vi "Forebrain.vi"() -> ()   [LabVIEW 2012]
doc: "This VI contrains the Forebrain within the Olin Robot Architecture. It must be run first to load the appropriate mission definition files. It contains a finite state machine built around a tabbed Operator interface that will guide an operator through the startup, run shutdown mission sequence. After running it, run the Midbrain and Hindbrain VIS."
panel:
  out "return count":u32
  out "error out":errorcluster
  in  "error in 2":errorcluster
  out "Desired \nVelocity":i16=5
  out "Local\nHeading":i16=90
  out "Ycurrent":dbl format="%#_3g"
  out "Xcurrent":dbl format="%#_3g"
  out "Ystart":dbl
  out "Xstart":dbl
  in  "error in":errorcluster
  out "Robot Live":bool
  in  "E-Stop":bool
  in  "Tab":T1(tab)
  out "MissionTime (Min)":dbl(knob) scale=0.0..10.0
  out "LidarDist":i16
  out "IR Index":i32
  out "BatteryLevel":dbl(slide) scale=6.0..9.0
  out "String Received":string
  out "Send String":string="$B^"
  in  "VISA resource name":refnum<visa-resource-name>="COM10"
  in  "Mode":i16 min=0 max=99 step=1
  in  "Desired Vel":i16(slide) scale=-9.0..9.0
  in  "Local Head":i16(slide) scale=-180.0..180.0
  out "StartMissionMap":picture
  out "MapDARCheck":picture
  in  "RunRobot":bool
  in  "Tug letter":string="G"
  out "Tug X":i32
  out "Tug Y":i32
  out "Tug H":i32
  out "BS Time Out?":bool
  out "Buoy locations":cluster{"regular expression":string, i32, i32}[](array[cluster])
  out "Valid ?":bool
  out "Battery\nVolts":i16
  out "Base Station data rec'd":string
  out "udp rate":bool
  out "CollisionWarning":bool
  out "DebugMapDAR":picture
  in  "MapDAR Control":T2={"NumberOfBeams"=180, "SensorRange"=500.0, "Noise (0.1 to 1)"=0.0} {"Noise (0.1 to 1)" min=0.0 max=1.0 step=0.1; "SensorRange" min=500.0 max=1500.0 step=100.0; "NumberOfBeams" min=36 max=360 step=2}
  out "MapDAR Data (r:pixel b:degrees)":cluster{"Range":dbl, "Bearing":dbl}[](array[cluster])
  in  "Stop DebugSENSE":bool
  out "MissionMap":picture
  out "Tug position":T3
  out "initialized MDF":T4(array[cluster])
  out "Way Point Index":i32
  out "InitialWaypoint":cluster{"X":i16, "Y":i16}
  in  "Pen Color":u32(colorbox)=15671808
  in  "Select Pen Attributes":T5={"Width"=1, "Style"=enum."Solid"}
  out "Draw??":bool
  in  "WhereAmI?FromBase":T6
  out "(xr,yr)":cluster{"X":dbl, "Y":dbl}
  in  "RobotPosition":T3 {"xrobot" min=0.0 max=1177.0 step=10.0; "yrobot" min=0.0 max=850.0 step=10.0; "heading" min=0.0 max=7.0 step=0.1}
  out "MDF_Original":T4(array[cluster])
  out "WhatAroundMeMap?":cluster{"T":dbl, "Range":dbl, "Bearing":dbl}[](array[cluster])
  out "WayPointAct":dbl[](array[numeric])
  out "SteerAngle":dbl
  out "MissionDefFile":picture
  out "MDF":T4(array[cluster])
  in  "Select Your Behavior":T7(ring)
  out "No. of Waypoints":i32
  in  "Exit Planning":bool
  in  "BoatSpeed for Leg":dbl(slide) min=-9.0 max=9.0 step=1.0 scale=-9.0..9.0
  out "BuildMDF":bool
  out "WayPoint Position":cluster{"X":i32, "Y":i32}
  out "Send String to NXT":string="$B^"
  in  "Behavior Command":T7(ring)
  out "CollisionLight":bool
  out "Where? Manual":T6
  out "ActManual":bool
  in  "Manual Heading":i16(knob) min=-179 max=180 step=5 scale=180.0..-180.0
  out "MWhat?":bool
  out "Where? 2":bool
  out "How? 2":bool
  in  "ManualModeStop":bool
  out "ManualModeMapDAR":picture
  out "ManualMissionMap":picture
  out "Battery":dbl(slide) scale=0.0..8.0
  in  "Manual Vel":dbl(slide) min=-6.0 max=6.0 step=1.0 scale=-6.0..6.0
  out "MissionTime":dbl(knob) scale=0.0..10.0
  out "Heading":cluster{dbl, dbl}(knob)={0.0, 34.390870865624734} scale=180.0..-179.0 scale format="%#_3g"
  out "Speed":i16(knob) scale=-6.0..6.0
  out "Current Behavior":T7(ring)
  out "Robot Position":cluster{"X":dbl, "Y":dbl} {"X" format="%#_3g"; "Y" format="%#_3g"}
  out "Ready":bool
  in  "Pause":bool
  in  "Rerun MDF":bool
  out "CollisionLight 2":bool
  out "Act":bool
  out "Neo-C":bool
  out "How?":bool
  out "What?":bool
  out "A Heading":cluster{dbl, dbl}(knob)={0.0, 34.390870865624734} scale=180.0..-180.0
  out "A Speed":dbl(knob) scale=-9.0..9.0
  out "AutoBattery":dbl(slide) scale=0.0..8.0
  out "AutoModeLIDAR":picture
  out "AutoMissionMap":picture
  in  "RunAutoMode":bool
  out "MissionTimeAuto":dbl(knob) scale=0.0..60.0
  out "Where?":bool
  # "To run\nrobot,\nclick\narrow\nabove\n\nRun Robot button must be on"
  # "Operation Directions\n\n1)Click on Startup&\nShutdown tab.\n2) Click on Run \nArrow on menubar.\nRun Forebrain,\nvis from the project\nexplorer.\n3) Select a mssion \nmap file when asked.\n4) Check robot is \nfully operational on\nStartup tab.\n5) Debug with debug\ntabs as required.\n6) Select ManualMode\ntab and test drive \nrobot.\n7) Select PlanMission\ntab and set up \nmission.\n8) Go to AutoMode\ntab and run mission."
  # "Turns off drive\nmotors"
  # "Enter Olin Test  Pool"
  # "Xbee Com Port"
  # "xBee\"Send String\" (mode, desired velocity, local heading)"
  # "(Type in Tug Letter  L T G P  (look at boat cradle)"
  # "Should be on to\nrun"
  # "BoatG,X,Y,H,BoatT,X,Y,H,BoatP,X,Y.H,BoatL,X,Y,H,BuoyA,X,Y,BuoyB,X,Y,BuoyC,X,Y,BuoyD,X,Y,Time(hours,Min,Sec)"
  # "To stop  program \nturn off here"
  # "Use this tab\nto explore\nLIDAR\ndata and \noperation"
  # "Set\nNumberOfBeams\nSensorRange\nNoise\nto\nview\nsimulated\nsensor\ndata"
  # "Turn Debug Sim \nto leave this\ntab--->"
  # "This tab will auto\nreturn to Startup \nin 2 seconds"
  # "Clean up interface and make more useful for debugging behaviors"
  # "Build out interface and make more useful for debugging act"
  # "This tab will auto\nreturn to Startup \nin 2 seconds"
  # "Directions:\n1) Select Robot Behavior for each mission leg.\n2) Select Robot Speed for leg.\n3) Click on robots current location for first waypoint.\n4) Hold down button and drag to next\nwaypoint. Click on next leg waypoint.\n5) Hold mouse button down and drag to \nnext waypoint. \n6) Click on next waypoint. Repeat for full mission.\n7) MDF will store up to 20 waypoints."
  # "Remember to\nset boat\nleg speed !"
  # "Please Adjust Scroll Barrs in Tug Off Mode to Prevent  Extra Lines Being Drawn"
  # "\"Send String\" (mode, desired velocity, local heading)"
  # "Press to stop and return to StartUp"
  # "Open MidBrain\nArbiter to see\nBrain Waves"
  # "AutoMode\nAutomatically \nReturns to \nStartUp Mode"
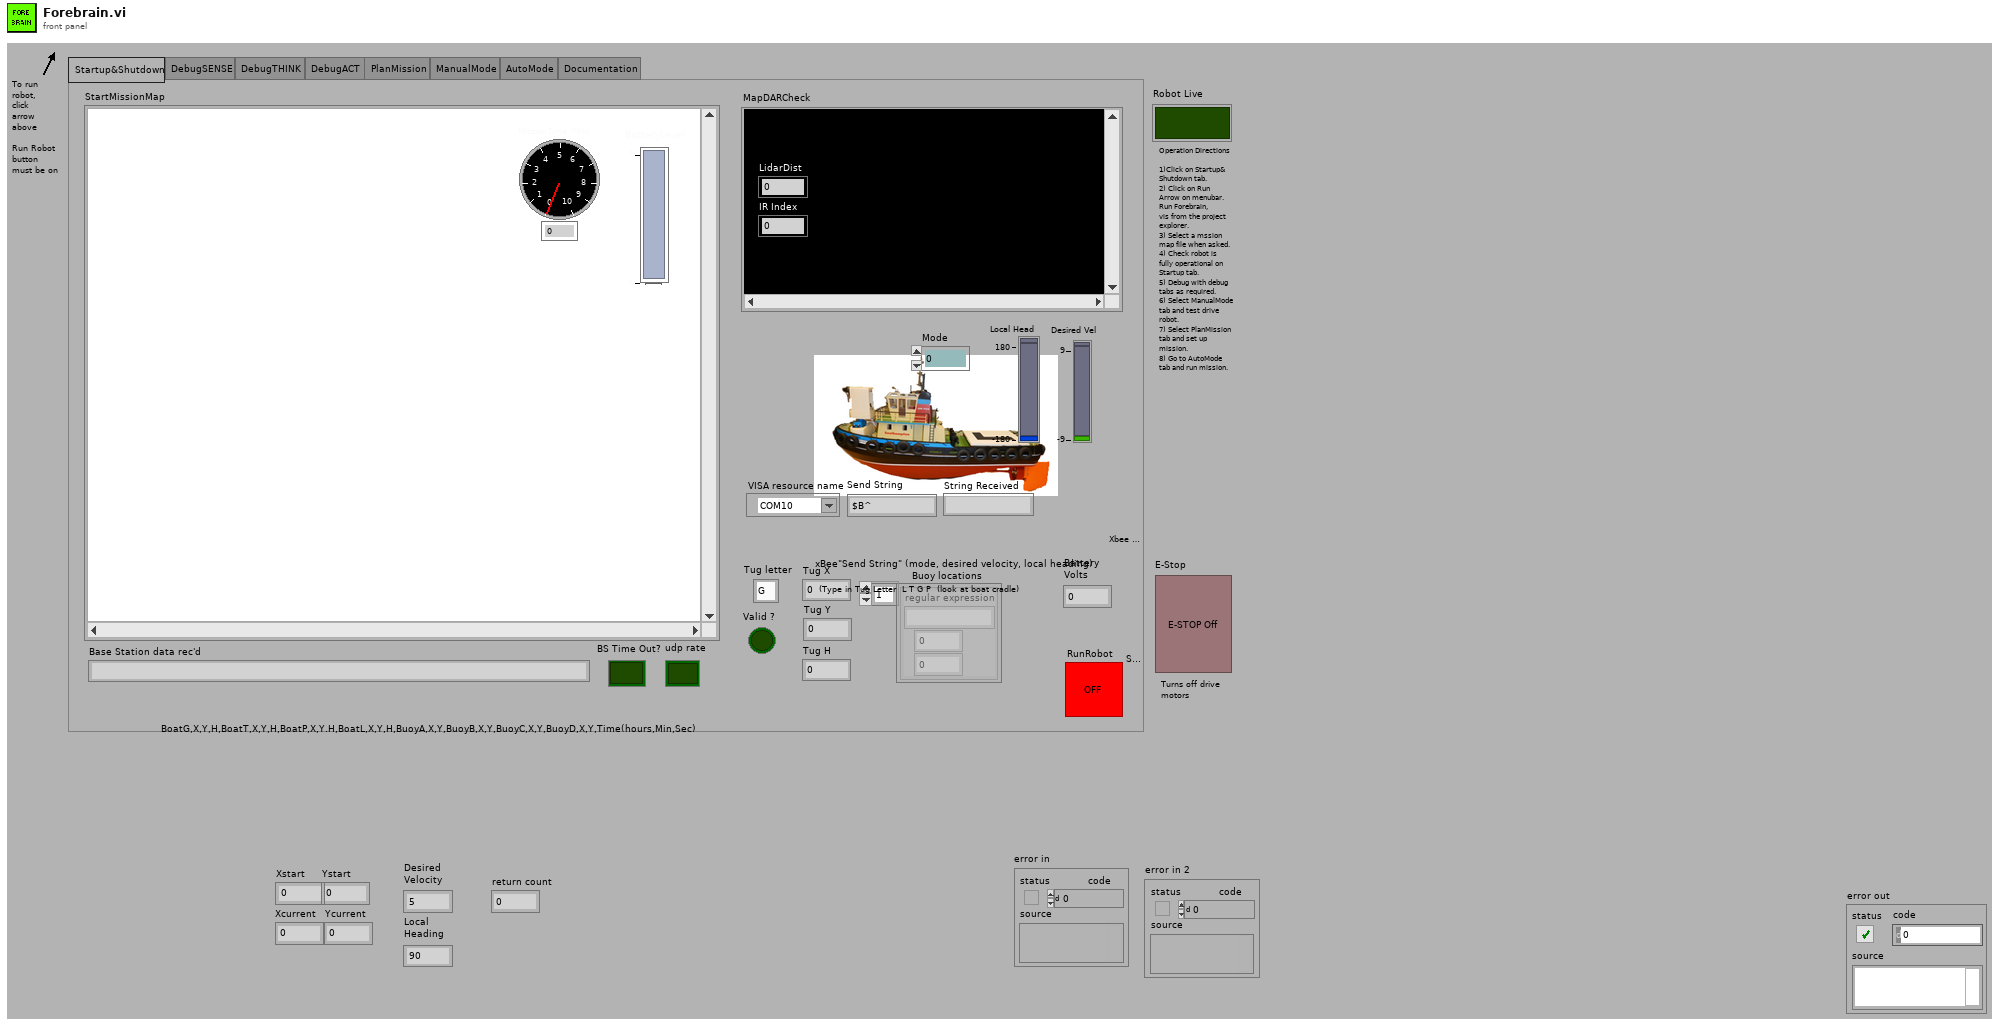
[diagram p1: front panel]
types:
  T1 = enum32{"Startup&Shutdown", "DebugSENSE", "DebugTHINK", "DebugACT", "PlanMission", "ManualMode", "AutoMode", "Documentation"}
  T2 = cluster{"NumberOfBeams":i32, "SensorRange":dbl, "Noise (0.1 to 1)":dbl}
  T3 = cluster{"xrobot":dbl, "yrobot":dbl, "heading":dbl}
  T4 = cluster{"Status":enum16{"Past", "Current", "Future"}, "x":dbl, "y":dbl, "z":dbl, "Vel":dbl, "Dwell Time":dbl, "BehCom":enum16{"Tug Off", "Manual Mode", "Goto WayPoint", "Back Up", "Circle", "Left Wall Follow", "Right Wall Follow", "Hunt"}, "Expand1":dbl, "Expand2":dbl, "Expand3":dbl}[]
  T5 = cluster{"Width":u16, "Style":enum32{"Solid", "Dash", "Dot", "DashDot", "DashDotDot"}}
  T6 = cluster{"T":dbl, "X":dbl, "Y":dbl, "Direction":dbl}
  T7 = enum16{"Tug Off", "Manual Mode", "Goto WayPoint", "Back Up", "Circle", "Left Wall Follow", "Right Wall Follow", "Hunt"}
  T8 = cluster{"VelCom":dbl, "BehCom":enum16{"OpenFieldTransit", "P-WallFollow", "S-WallFollow", "LaneFollow", "ManualMode"}}
  T9 = typedef "IMAQ Image.ctl" = refnum<image>
  T10 = typedef "imagedata.ctl" = cluster{"image type":i32, "image depth":i32, "image":u8[], "mask":u8[], "colors":u32[], "Rectangle":cluster{"left":i16, "top":i16, "right":i16, "bottom":i16}}
  T11 = cluster{"Status":enum16{"Past", "Current", "Future"}, "x":dbl, "y":dbl, "z":dbl, "Vel":dbl, "Dwell Time":dbl, "BehCom":enum16{"Tug Off", "Manual Mode", "Goto WayPoint", "Back Up", "Circle", "Left Wall Follow", "Right Wall Follow", "Hunt"}, "Expand1":dbl, "Expand2":dbl, "Expand3":dbl}
  T12 = typedef "LVMouseTypeDef.ctl" = cluster{"Mouse Position":cluster{"X":i32, "Y":i32}, "Mouse Modifiers":cluster{"Button Down":bool, "Shift Mod":bool, "Menu Mod":bool, "Option Mod":bool}}
  T13 = cluster{"regular expression":string, i32, i32, i32}
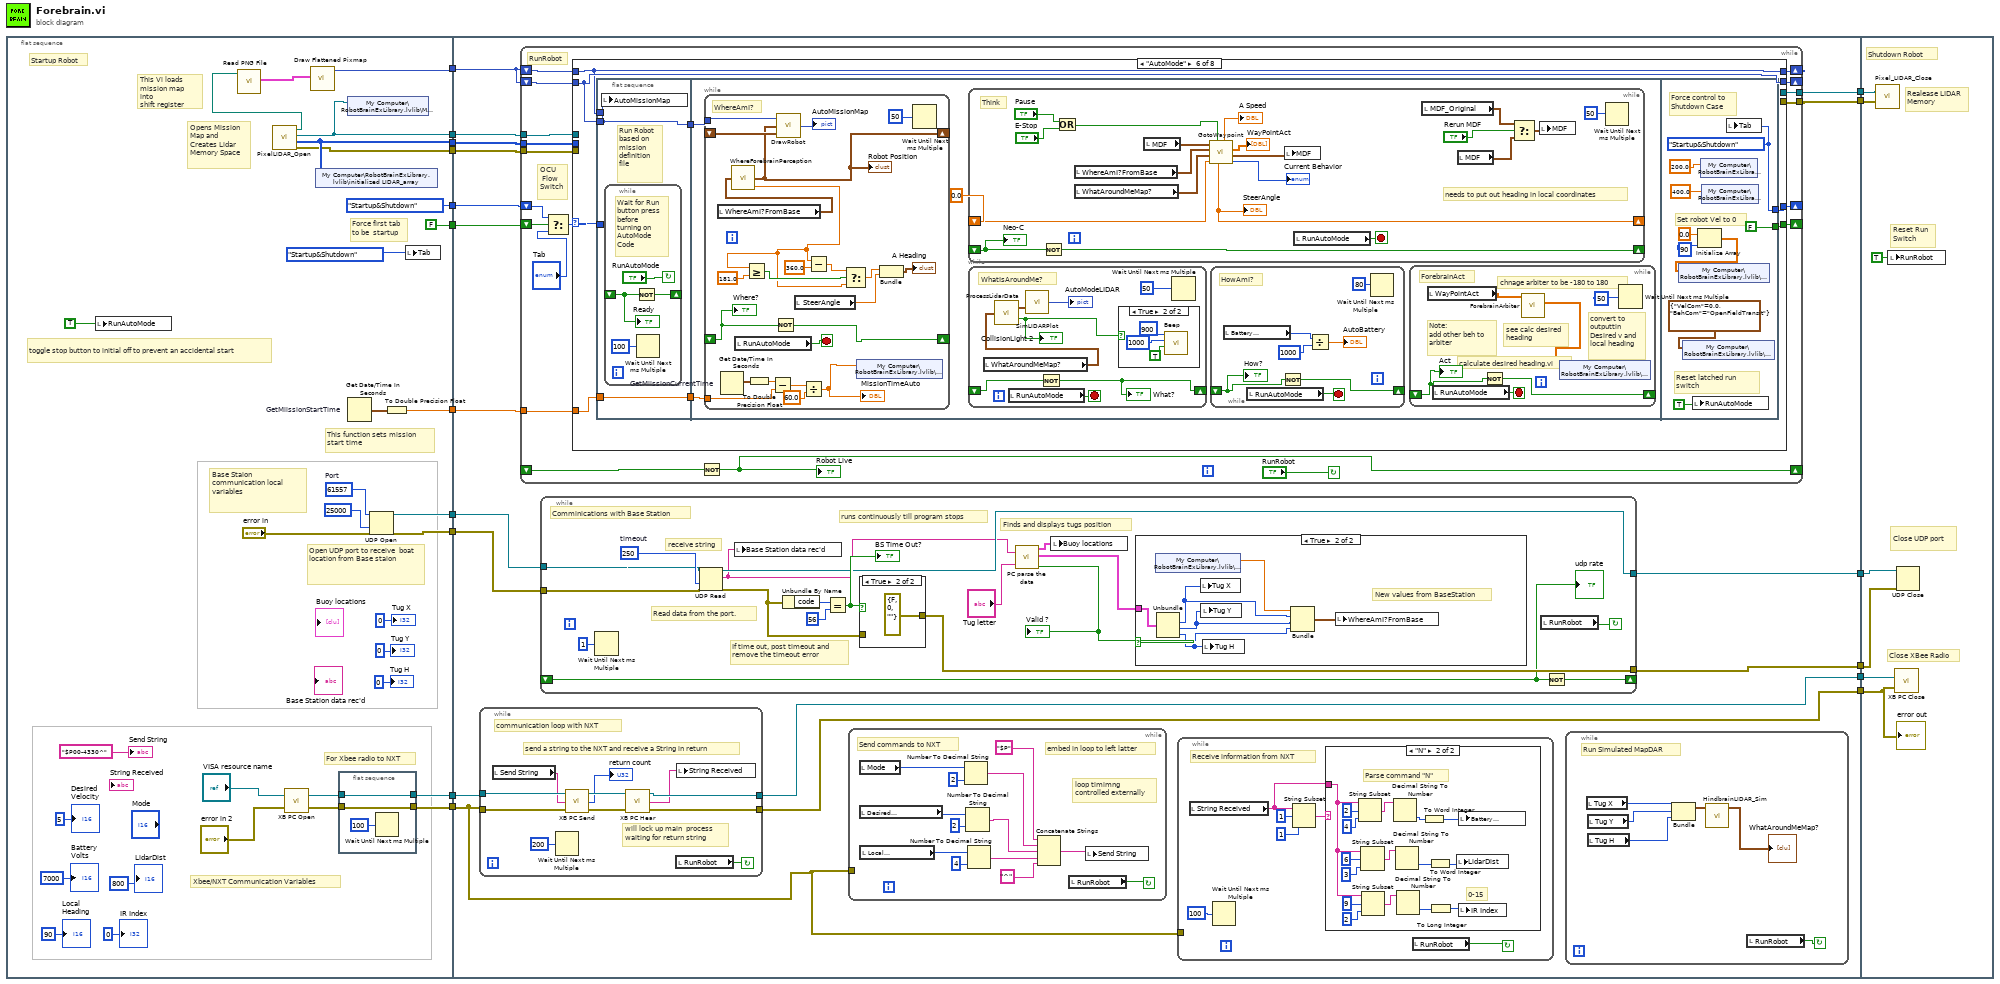
[diagram p0: block diagram]
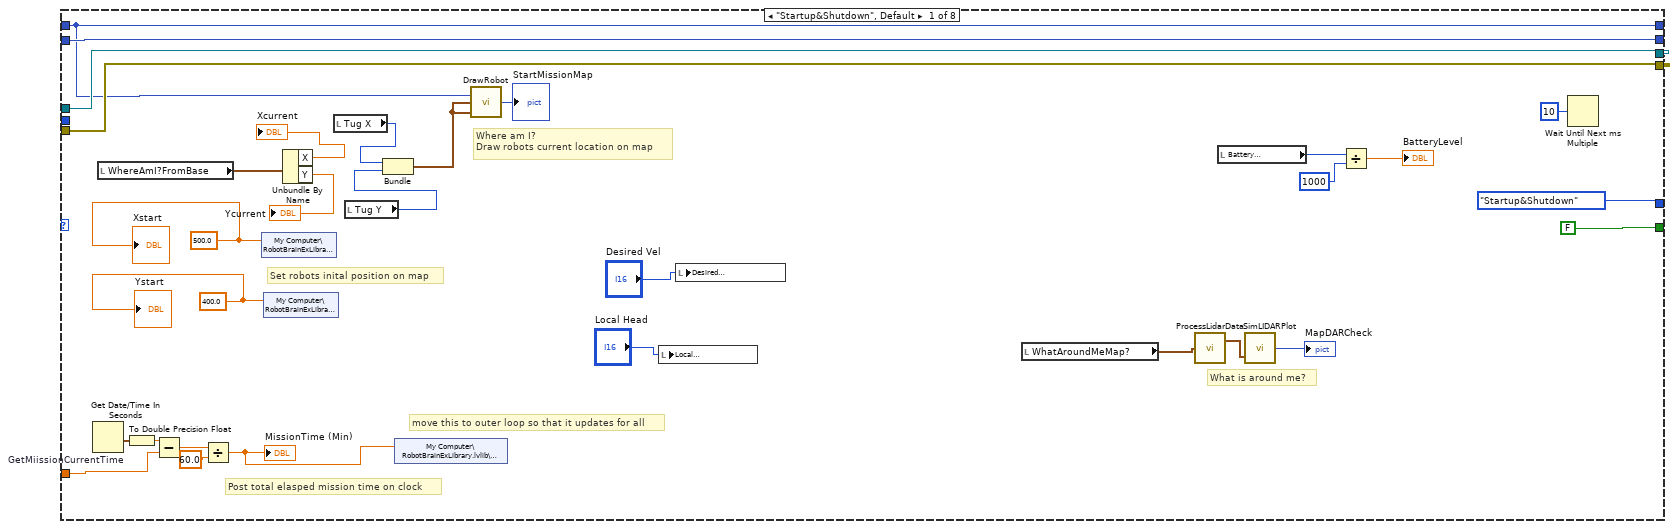
[diagram p5: hidden frame]
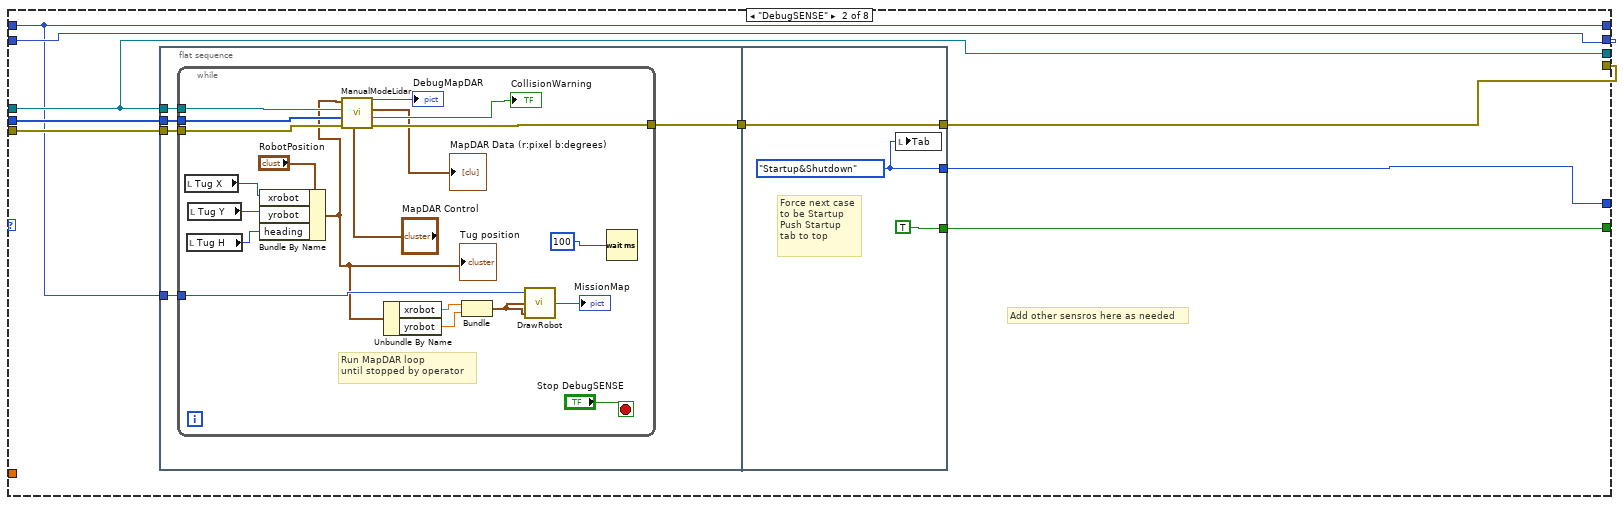
[diagram p6: hidden frame]
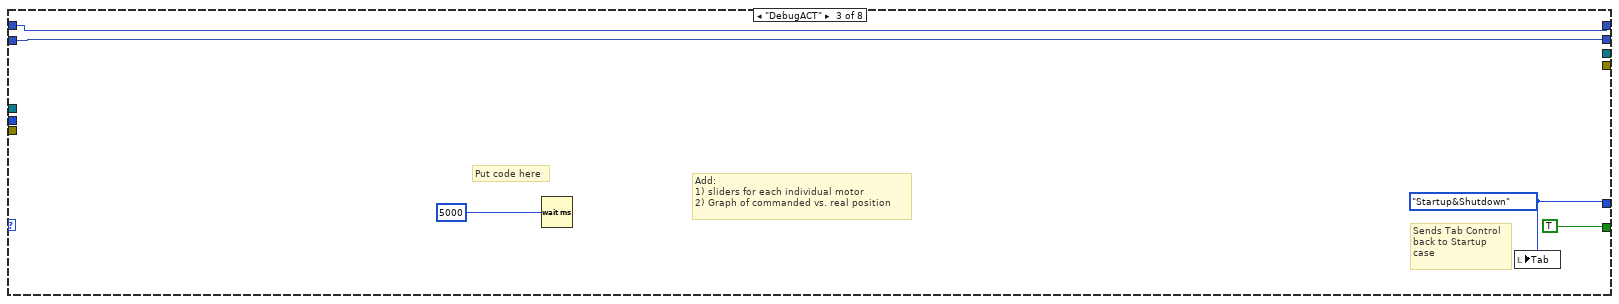
[diagram p7: hidden frame]
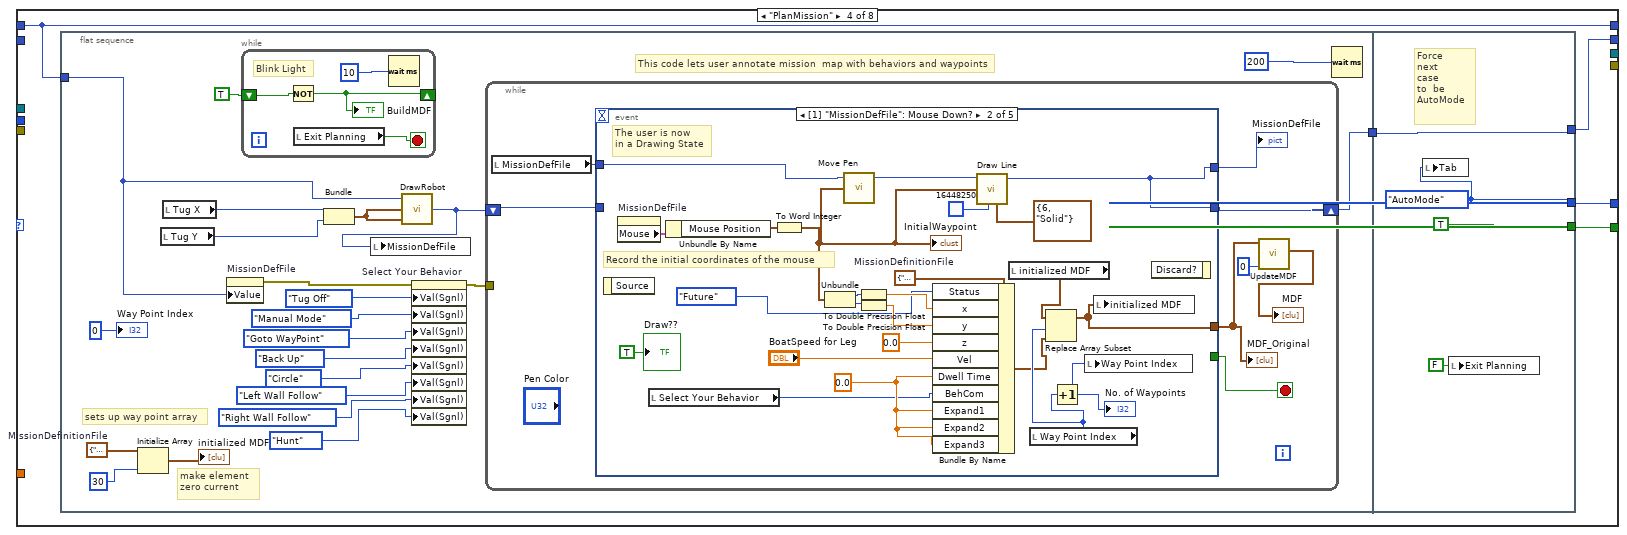
[diagram p8: hidden frame]
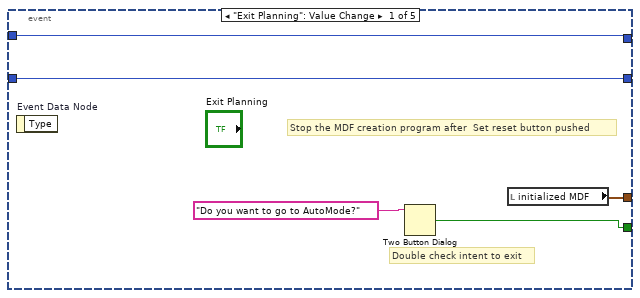
[diagram p9: hidden frame]
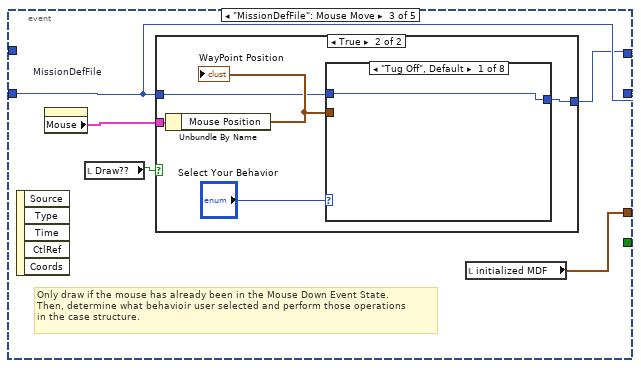
[diagram p10: hidden frame]
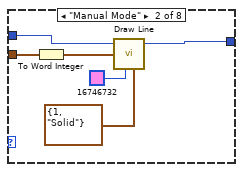
[diagram p12: hidden frame]
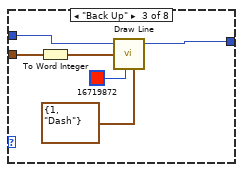
[diagram p13: hidden frame]
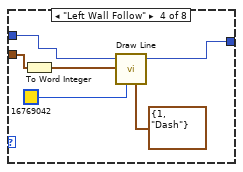
[diagram p14: hidden frame]
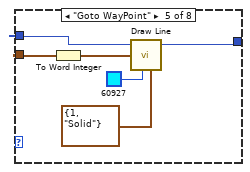
[diagram p15: hidden frame]
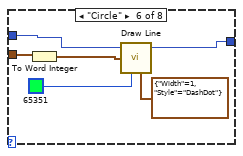
[diagram p16: hidden frame]
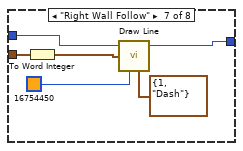
[diagram p17: hidden frame]
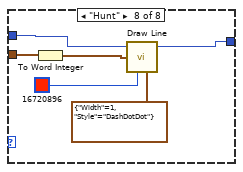
[diagram p18: hidden frame]
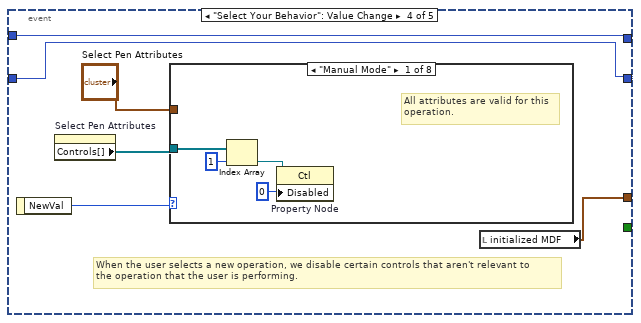
[diagram p19: hidden frame]
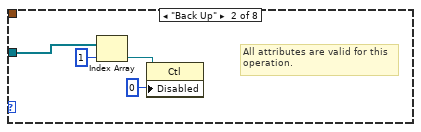
[diagram p20: hidden frame]
diagram:
  n1 = flat-sequence {
    tunnel: [w48] -> w17
    tunnel: [w47] -> w16
    tunnel: [w44] -> w15
    tunnel: [w46] -> w14
    tunnel: [w45] -> w13
    tunnel: [FALSE ("RunAutoMode")] -> w10
    tunnel: [T1."Startup&Shutdown" ("Tab")] -> w9
    tunnel: [w31] -> w8
    tunnel: [w30] -> w7
    tunnel: [w19] -> w6
    tunnel: [w18] -> w5
    tunnel: w17 -> [w69]
    tunnel: w16 -> [w68]
    tunnel: w15 -> [w67]
    tunnel: w14 -> [w66]
    tunnel: w13 -> [w65]
    tunnel: [w64] -> w12
    tunnel: [w63] -> w11
    tunnel: w10 -> [w62]
    tunnel: w9 -> [w61]
    tunnel: w8 -> [w56]
    tunnel: w7 -> [w55]
    tunnel: w6 -> [w60]
    tunnel: w5 -> [w57]
    tunnel: [w59] -> w4
    tunnel: [w58] -> w3
    tunnel: [w54] -> w2
    tunnel: [w53] -> w1
    tunnel: w12 -> [w586]
    tunnel: w11 -> [w585]
    tunnel: w4 -> [w584]
    tunnel: w3 -> [w583]
    tunnel: w2 -> [w582]
    tunnel: w1 -> [w581]
    frame #0 {
      w37 = u16 61557  # Port
      # "For Xbee radio to NXT"
      # "Xbee/NXT Communication Variables"
      # "Base Staion communication local variables"
      # "Open UDP port to receive  boat location from Base staion"
      # "Force first tab\nto be  startup"
      # "toggle stop button to initial off to prevent an accidental start"
      # "Opens Mission\nMap and\nCreates Lidar\nMemory Space"
      # "This function sets mission \nstart time"
      # "This Vi loads\nmission map into \nshift register"
      # "Startup Robot"
      n2 = local write "RunAutoMode"(TRUE ("RunAutoMode")) -> ()
      n3 = call "PixelLIDAR_Open.vi"() -> ("error out"=w45:errorcluster, "initialized LIDAR\narray"=w46:i32[], "MDF Image"=w44:T9, "MissionMap"=w39:path)  [unwired: 2 in]
      n4 = call <vilib>:"Read PNG File.vi"("path to PNG file"=w39) -> ("image data"=w38:T10)  [unwired: 8 in, 2 out]
      n5 = call "XB PC Open.vi"("error in (no error)"="error in 2", "VISA resource name"="VISA resource name") -> ("error out"=w22:errorcluster, "VISA resource name out"=w23:refnum<visa-resource-name>)
      n6 = call <vilib>:"Draw Flattened Pixmap.vi"("image data"=w38) -> ("new picture"=w47:picture)  [unwired: 8 in]
      n7 = shared-variable "My Computer\\RobotBrainExLibrary.lvlib\\initialized LIDAR_array"(w46) -> ()  [unwired: 1 in, 1 out]
      n8 = flat-sequence {
        tunnel: w23 -> [w50]
        tunnel: w22 -> [w51]
        tunnel: [w51] -> w18
        tunnel: [w50] -> w19
        frame #0 {
          n9 = Wait Until Next ms Multiple(millisecond multiple=u32 100) -> ()  [unwired: 1 out]
        }
      }
      n10 = shared-variable "My Computer\\RobotBrainExLibrary.lvlib\\MDF Image"(w44) -> ()  [unwired: 1 in, 1 out]
      n11 = Get Date/Time In Seconds "GetMiissionStartTime"() -> (seconds since 1Jan1904=w49:timestamp)
      n12 = UDP Open(8:"error in", 9:25000 ("timeout ms (25000)"), 11:w37) -> (port=w31:refnum<k16>, 0:w30:errorcluster)  [unwired: 2 in, 1 out]
      n13 = To Double Precision Float(number=w49) -> (double precision float=w48:dbl)
      n14 = local write "Tab"(T1."Startup&Shutdown" ("Tab")) -> ()
      "Tug X" <- 0 ("Tug X")
      "Tug Y" <- 0 ("Tug Y")
      "Tug H" <- 0 ("Tug H")
      "Battery\nVolts" <- i16 7000 ("Battery\nVolts")
      "LidarDist" <- i16 800 ("Dist")
      "IR Index" <- 0 ("IR Index")
      "Local\nHeading" <- i16 90 ("Local\nHeading")
      "Desired \nVelocity" <- i16 5 ("Desired \nVelocity")
      "Send String" <- "$P00-4330^"
    }
    frame #1 {
      n15 = while {
        tunnel: w60 -> [w121]
        tunnel: w57 -> [w120]
        tunnel: [w117] -> w58
        tunnel: [w116] -> w59
        stop <- w115 continue-if-true
        # "will lock up main  process\nwaiting for return string"
        # "communication loop with NXT"
        # "send a string to the NXT and receive a String in return"
        n16 = local read "Send String"() -> (w113:string)
        n17 = Wait Until Next ms Multiple(millisecond multiple=u32 200) -> ()  [unwired: 1 out]
        n18 = call "XB PC Send.vi"("error in (no error)"=w120, "String"=w113, "VISA resource name"=w121) -> ("error out"=w119:errorcluster, "return count"=→"return count":u32, "VISA resource name out"=w118:refnum<visa-resource-name>)
        n19 = call "XB PC Hear.vi"("VISA resource name"=w118, "error in (no error)"=w119) -> ("VISA resource name out"=w116:refnum<visa-resource-name>, "String Received"=w112:string, "error out"=w117:errorcluster)
        n20 = local read "RunRobot"() -> (w115:bool)
        n21 = local write "String Received"(w112) -> ()
      }
      n22 = while {
        shift-right: [w148] -> _
        shift-left: _ -> [w165]
        shift-right: [w164] -> _
        shift-left: w61 -> [w163]
        shift-right: [w160] -> _
        shift-left: w62 -> [w159]
        tunnel: w69 -> [w158]
        shift-right: [w156] -> _
        shift-left: w68 -> [w157]
        shift-right: [w154] -> _
        shift-left: w68 -> [w155]
        tunnel: w67 -> [w153]
        tunnel: w66 -> [w152]
        tunnel: w65 -> [w151]
        tunnel: [w150] -> w64
        tunnel: [w149] -> w63
        stop <- "RunRobot" continue-if-true
        # "RunRobot"
        # "OCU\n Flow\nSwitch"
        n23 = Select(t=w163, s=w159, f="Tab") -> (s? t:f=w161:T1)
        n24 = case shown="\"AutoMode\"" w161 {
          selector: w161 -> [_ _ _ _ _ w484 _ _]
          tunnel: [T1."Startup&Shutdown" ("Tab") w201 w236 w243 w410 w485 T1."Startup&Shutdown" ("Tab") w579] -> w164
          tunnel: [FALSE ("s") w200 TRUE ("s") w242 w411 w483 FALSE ("s") TRUE ("s")] -> w160
          tunnel: w158 -> [w190 _ _ _ w408 w481 _ _]
          tunnel: w157 -> [w183 w197 w235 w239 w406 w478 w572 w577]
          tunnel: [w183 w197 w235 w239 w406 w478 w572 w577] -> w156
          tunnel: w155 -> [w189 w198 w234 _ w407 w480 w571 w576]
          tunnel: [w189 w198 w234 w240 w407 w480 w571 w576] -> w154
          tunnel: w153 -> [w188 w199 _ _ _ _ _ _]
          tunnel: w152 -> [_ w205 _ _ _ _ _ _]
          tunnel: w151 -> [w187 w204 _ _ _ _ _ _]
          tunnel: [w188 w199 _ _ _ _ _ _] -> w150
          tunnel: [w187 w203 _ _ _ _ _ _] -> w149
          frame "Startup&Shutdown", Default {
            w178 = 400.0 ("Ystart")
            w179 = 500.0 ("Xstart")
            # "move this to outer loop so that it updates for all"
            # "Where am I?\nDraw robots current location on map"
            # "Post total elasped mission time on clock"
            # "What is around me?"
            # "Set robots inital position on map"
            n25 = Get Date/Time In Seconds "GetMiissionCurrentTime"() -> (seconds since 1Jan1904=w194:timestamp)
            n26 = local read "WhereAmI?FromBase"() -> (w167:T6)
            n27 = To Double Precision Float(number=w194) -> (double precision float=w193:dbl)
            n28 = Subtract(x=w193, y=w190) -> (x-y=w192:dbl)
            n29 = Divide(x=w192, y=60.0) -> (x/y=w186:dbl)
            "MissionTime (Min)" <- w186
            n30 = shared-variable "My Computer\\RobotBrainExLibrary.lvlib\\Xstart"(w179) -> ()  [unwired: 1 in, 1 out]
            n31 = shared-variable "My Computer\\RobotBrainExLibrary.lvlib\\Ystart"(w178) -> ()  [unwired: 1 in, 1 out]
            n32 = Unbundle By Name(w167) -> ("X"=→"Xcurrent":dbl, "Y"=→"Ycurrent":dbl)
            n33 = local read "Tug X"() -> (w177:i32)
            n34 = local read "Tug Y"() -> (w176:i32)
            n35 = Bundle("Tug X"=w177, "Tug Y"=w176) -> (w182:cluster{"Tug X":i32, "Tug Y":i32})  [unwired: 1 in]
            n36 = shared-variable "My Computer\\RobotBrainExLibrary.lvlib\\MissionTime"(w186) -> ()  [unwired: 1 in, 1 out]
            n37 = call "DrawRobot.vi"("(xr,yr) old"=w182, "(xr,yr) new"=w182, "2D Picture"=w183) -> ("new picture"=→"StartMissionMap":picture)
            n38 = local write "Local\nHeading"("Local Head") -> ()
            n39 = local write "Desired \nVelocity"("Desired Vel") -> ()
            n40 = local read "WhatAroundMeMap?"() -> (w168:cluster{"T":dbl, "Range":dbl, "Bearing":dbl}[])
            n41 = call "ProcessLidarData.vi"("WhatAroundMe?MM"=w168) -> ("data array [mag, phase (deg)]"=w184:cluster{"magnitude":dbl, "phase":dbl}[])  [unwired: 1 out]
            n42 = local read "Battery\nVolts"() -> (w173:i16)
            n43 = call "SimLIDARPlot.vi"("data array [mag, phase (deg)]"=w184) -> ("SONAR"=→"MapDARCheck":picture)  [unwired: 1 in]
            n44 = Divide(x=w173, y=i16 1000) -> (x/y=→"BatteryLevel":dbl)
            n45 = Wait Until Next ms Multiple(millisecond multiple=u32 10) -> ()  [unwired: 1 out]
            "Xstart" <- w179
            "Ystart" <- w178
          }
          frame "DebugSENSE" {
            # "Add other sensros here as needed"
            n46 = flat-sequence {
              tunnel: w205 -> [w210]
              tunnel: w204 -> [w209]
              tunnel: w199 -> [w208]
              tunnel: [w207] -> w202
              tunnel: w197 -> [w206]
              tunnel: [w233] -> w203
              tunnel: w202 -> [w233]
              tunnel: [w232] -> w201
              tunnel: [TRUE ("s")] -> w200
              frame #0 {
                n47 = while {
                  tunnel: w210 -> [w230]
                  tunnel: w209 -> [w229]
                  tunnel: w208 -> [w228]
                  tunnel: [w227] -> w207
                  tunnel: w206 -> [w221]
                  stop <- "Stop DebugSENSE" stop-if-true
                  # "Run MapDAR loop\nuntil stopped by operator"
                  n48 = local read "Tug X"() -> (w215:i32)
                  n49 = local read "Tug H"() -> (w216:i32)
                  n50 = local read "Tug Y"() -> (w214:i32)
                  n51 = Bundle By Name(cluster="RobotPosition", "xrobot"=w215, "yrobot"=w214, "heading"=w216) -> (w212:T3)
                  "Tug position" <- w212
                  n52 = call "ManualModeLidar.vi"("LIDARControl"="MapDAR Control", "error in"=w229, "initialized \nsonar ray\narray"=w230, "MDF Image"=w228, "SubPosition"=w212) -> ("error out"=w227:errorcluster, "Collision\nWarning"=→"CollisionWarning":bool, "LIDAR Data (r:pixel b:degrees)"=→"MapDAR Data (r:pixel b:degrees)":cluster{"Range":dbl, "Bearing":dbl}[], "LIDAR"=→"DebugMapDAR":picture)  [unwired: 1 in]
                  n53 = Unbundle By Name(w212) -> ("xrobot"=w219:dbl, "yrobot"=w218:dbl)
                  n54 = Bundle("xrobot"=w219, "yrobot"=w218) -> (w211:cluster{"xrobot":dbl, "yrobot":dbl})  [unwired: 1 in]
                  n55 = call "DrawRobot.vi"("(xr,yr) old"=w211, "(xr,yr) new"=w211, "2D Picture"=w221) -> ("new picture"=→"MissionMap":picture)
                  n56 = Wait (ms)(milliseconds to wait=u32 100) -> ()  [unwired: 1 out]
                }
              }
              frame #1 {
                w232 = T1."Startup&Shutdown" ("Tab")
                # "Force next case\nto be Startup\nPush Startup\ntab to top"
                n57 = local write "Tab"(w232) -> ()
              }
            }
          }
          frame "DebugACT" {
            w236 = T1."Startup&Shutdown" ("Tab")
            # "Add:\n1) sliders for each individual motor\n2) Graph of commanded vs. real position"
            # "Put code here"
            # "Sends Tab Control\nback to Startup\ncase"
            n58 = Wait (ms)(milliseconds to wait=u32 5000) -> ()  [unwired: 1 out]
            n59 = local write "Tab"(w236) -> ()
          }
          frame "PlanMission" {
            n60 = flat-sequence {
              tunnel: [w264] -> w241
              tunnel: w239 -> [w257]
              tunnel: [w404] -> w243
              tunnel: [TRUE ("s")] -> w242
              tunnel: w241 -> [w403]
              tunnel: [w403] -> w240
              frame #0 {
                w255 = T11 {"Status"=enum."Future", "x"=0.0, "y"=0.0, "z"=0.0, "Vel"=0.0, "Dwell Time"=0.0, "BehCom"=enum."Tug Off", "Expand1"=0.0, "Expand2"=0.0, "Expand3"=0.0}  # MissionDefinitionFile
                # "make element \nzero current"
                # "sets up way point array"
                # "This code lets user annotate mission  map with behaviors and waypoints"
                n61 = Initialize Array ("Initialize WaypointArray")(w255, 30 ("dimension size")) -> (→"initialized MDF":T4)
                n62 = local read "Tug Y"() -> (w252:i32)
                n63 = local read "Tug X"() -> (w253:i32)
                n64 = property on="MissionDefFile" class="Pict"("Value"=w257) -> (error out=w262:errorcluster)  [unwired: 2 in, 1 out]
                n65 = while {
                  shift-right: [w268] -> _
                  shift-left: TRUE -> [w269]
                  stop <- w267 stop-if-true
                  # "Blink Light"
                  n66 = Not(x=w269) -> (.not. x?=w268:bool)
                  "BuildMDF" <- w268
                  n67 = local read "Exit Planning"() -> (w267:bool)
                  n68 = Wait (ms)(milliseconds to wait=u32 10) -> ()  [unwired: 1 out]
                }
                n69 = Bundle("Tug X"=w253, "Tug Y"=w252) -> (w258:cluster{"Tug X":i32, "Tug Y":i32})  [unwired: 1 in]
                n70 = call "DrawRobot.vi"("(xr,yr) old"=w258, "(xr,yr) new"=w258, "2D Picture"=w257) -> ("new picture"=w256:picture)
                n71 = local write "MissionDefFile"(w256) -> ()
                n72 = property on="Select Your Behavior" class="Enum (strict)"(error in=w262, "Val(Sgnl)"=T7."Tug Off" ("Value (Signaling)"), "Val(Sgnl)"=T7."Manual Mode" ("Value (Signaling)"), "Val(Sgnl)"=T7."Goto WayPoint" ("Value (Signaling)"), "Val(Sgnl)"=T7."Back Up" ("Value (Signaling)"), "Val(Sgnl)"=T7."Circle" ("Value (Signaling)"), "Val(Sgnl)"=T7."Left Wall Follow" ("Value (Signaling)"), "Val(Sgnl)"=T7."Right Wall Follow" ("Value (Signaling)"), "Val(Sgnl)"=T7."Hunt" ("Value (Signaling)")) -> (error out=w263:errorcluster)  [unwired: 1 in, 1 out]
                n73 = while {
                  shift-right: [w276] -> w264
                  shift-left: w256 -> [w277]
                  tunnel: w263 -> [_]
                  stop <- w275 stop-if-true
                  n74 = local read "MissionDefFile"() -> (w274:picture)
                  n75 = event shown="[1] \"MissionDefFile\": Mouse Down?" {
                    selector: _ -> [_ _ _ _ _]
                    dyn-events: _ -> [_ _ _ _ _]
                    timeout: _ -> [_ _ _ _ _]
                    tunnel: [w280 w288 w308 w361 w399] -> w276
                    tunnel: w277 -> [w280 _ w308 w361 _]
                    tunnel: [w281 _ _ _ _] -> w275
                    tunnel: [w279 w303 w309 w363 w400] -> w271
                    tunnel: w274 -> [w278 w289 _ w362 w399]
                    tunnel: [w278 w288 w307 w362 w399] -> w273
                    event "Exit Planning": Value Change {
                      # "Double check intent to exit"
                      # "Stop the MDF creation program after  Set reset button pushed"
                      n76 = event-data "Event Data Node"() -> ()  [unwired: 1 in, 1 out]
                      n77 = Two Button Dialog(message="Do you want to go to AutoMode?") -> (T button?=w281:bool)  [unwired: 2 in]
                      n78 = local read "initialized MDF"() -> (w279:T4)
                    }
                    event "MissionDefFile": Mouse Down? {
                      w287 = T11 {"Status"=enum."Future", "x"=0.0, "y"=0.0, "z"=0.0, "Vel"=0.0, "Dwell Time"=0.0, "BehCom"=enum."Tug Off", "Expand1"=0.0, "Expand2"=0.0, "Expand3"=0.0}  # MissionDefinitionFile
                      w297 = 0.0 ("Dwell Time")
                      # "Record the initial coordinates of the mouse"
                      # "The user is now\nin a Drawing State"
                      n79 = event-data() -> ()  [unwired: 1 in, 1 out]
                      n80 = property on="MissionDefFile" class="Pict"() -> ("Mouse"=w306:T12)  [unwired: 2 in, 2 out]
                      n81 = local read "Select Your Behavior"() -> (w284:T7)
                      n82 = Unbundle By Name(w306) -> ("Mouse Position"=w304:cluster{"X":i32, "Y":i32})
                      n83 = To Word Integer(number=w304) -> (16bit integer=w292:cluster{"X":i16, "Y":i16})
                      "InitialWaypoint" <- w292
                      n84 = Unbundle(w292) -> ("X"=w301:i16, "Y"=w300:i16)
                      n85 = call <vilib>:"Move Pen.vi"("new position"=w292, "picture"=w289) -> ("new picture"=w293:picture)  [unwired: 3 in]
                      n86 = To Double Precision Float(number=w301) -> (double precision float=w299:dbl)
                      n87 = To Double Precision Float(number=w300) -> (double precision float=w298:dbl)
                      n88 = Bundle By Name(cluster=w287, "Status"=enum16{"Past", "Current", "Future"}."Future", "x"=w299, "y"=w298, "z"=0.0, "Vel"="BoatSpeed for Leg", "Dwell Time"=w297, "BehCom"=w284, "Expand1"=w297, "Expand2"=w297, "Expand3"=w297) -> (w283:T11)
                      n89 = call <vilib>:"Draw Line.vi"("picture"=w293, "end point"=w292, "color(black)"=u32 16448250, "pen"=T5 {"Width"=6, "Style"=enum."Solid"}) -> ("new picture"=w288:picture)  [unwired: 5 in]
                      n90 = local read "initialized MDF"() -> (w302:T4)
                      n91 = local read "Way Point Index"() -> (w285:i32)
                      n92 = Replace Array Subset(array=w302, new element=w283, index=w285) -> (w303:T4)
                      n93 = Increment(x=w285) -> (x+1=w305:i32)
                      "No. of Waypoints" <- w305
                      n94 = local write "Way Point Index"(w305) -> ()
                      n95 = local write "initialized MDF"(w303) -> ()
                      n96 = event-data() -> ()  [unwired: 2 in, 1 out]
                      "Draw??" <- TRUE ("Draw??")
                    }
                    event "MissionDefFile": Mouse Move {
                      # "Only draw if the mouse has already been in the Mouse Down Event State.\nThen, determine what behavioir user selected and perform those operations\nin the case structure."
                      n97 = event-data() -> ()  [unwired: 1 in, 5 out]
                      n98 = property on="MissionDefFile" class="Pict"() -> ("Mouse"=w311:T12)  [unwired: 2 in, 2 out]
                      n99 = local read "Draw??"() -> (w310:bool)
                      n100 = case shown="True" w310 {
                        tunnel: w311 -> [_ w317]
                        tunnel: w308 -> [w312 w313]
                        tunnel: [w312 w314] -> w307
                        frame False {
                        }
                        frame True {
                          n101 = Unbundle By Name(w317) -> ("Mouse Position"=w315:cluster{"X":i32, "Y":i32})
                          "WayPoint Position" <- w315
                          n102 = case shown="\"Tug Off\", Default" "Select Your Behavior" {
                            tunnel: w315 -> [_ w323 w329 w332 w338 w343 w349 w355]
                            tunnel: [w318 w324 w330 w334 w337 w344 w350 w356] -> w314
                            tunnel: w313 -> [w318 w322 w326 w335 w339 w345 w351 w357]
                            frame "Tug Off", Default {
                            }
                            frame "Manual Mode" {
                              n103 = To Word Integer(number=w323) -> (16bit integer=w319:cluster{"X":i16, "Y":i16})
                              n104 = call <vilib>:"Draw Line.vi"("picture"=w322, "end point"=w319, "color(black)"=u32 16746732, "pen"=T5 {"Width"=1, "Style"=enum."Solid"}) -> ("new picture"=w324:picture)  [unwired: 5 in]
                            }
                            frame "Back Up" {
                              n105 = To Word Integer(number=w329) -> (16bit integer=w325:cluster{"X":i16, "Y":i16})
                              n106 = call <vilib>:"Draw Line.vi"("picture"=w326, "end point"=w325, "color(black)"=u32 16719872, "pen"=T5 {"Width"=1, "Style"=enum."Dash"}) -> ("new picture"=w330:picture)  [unwired: 5 in]
                            }
                            frame "Left Wall Follow" {
                              n107 = To Word Integer(number=w332) -> (16bit integer=w333:cluster{"X":i16, "Y":i16})
                              n108 = call <vilib>:"Draw Line.vi"("picture"=w335, "end point"=w333, "color(black)"=u32 16769042, "pen"=T5 {"Width"=1, "Style"=enum."Dash"}) -> ("new picture"=w334:picture)  [unwired: 5 in]
                            }
                            frame "Goto WayPoint" {
                              n109 = To Word Integer(number=w338) -> (16bit integer=w340:cluster{"X":i16, "Y":i16})
                              n110 = call <vilib>:"Draw Line.vi"("picture"=w339, "end point"=w340, "color(black)"=u32 60927, "pen"=T5 {"Width"=1, "Style"=enum."Solid"}) -> ("new picture"=w337:picture)  [unwired: 5 in]
                            }
                            frame "Circle" {
                              n111 = To Word Integer(number=w343) -> (16bit integer=w348:cluster{"X":i16, "Y":i16})
                              n112 = call <vilib>:"Draw Line.vi"("picture"=w345, "end point"=w348, "color(black)"=u32 65351, "pen"=T5 {"Width"=1, "Style"=enum."DashDot"}) -> ("new picture"=w344:picture)  [unwired: 5 in]
                            }
                            frame "Right Wall Follow" {
                              n113 = To Word Integer(number=w349) -> (16bit integer=w354:cluster{"X":i16, "Y":i16})
                              n114 = call <vilib>:"Draw Line.vi"("picture"=w351, "end point"=w354, "color(black)"=u32 16754450, "pen"=T5 {"Width"=1, "Style"=enum."Dash"}) -> ("new picture"=w350:picture)  [unwired: 5 in]
                            }
                            frame "Hunt" {
                              n115 = To Word Integer(number=w355) -> (16bit integer=w358:cluster{"X":i16, "Y":i16})
                              n116 = call <vilib>:"Draw Line.vi"("picture"=w357, "end point"=w358, "color(black)"=u32 16720896, "pen"=T5 {"Width"=1, "Style"=enum."DashDotDot"}) -> ("new picture"=w356:picture)  [unwired: 5 in]
                            }
                          }
                        }
                      }
                      n117 = local read "initialized MDF"() -> (w309:T4)
                    }
                    event "Select Your Behavior": Value Change {
                      # "When the user selects a new operation, we disable certain controls that aren't relevant to\nthe operation that the user is performing."
                      n118 = event-data() -> ("NewVal"=w366:T7)  [unwired: 1 in]
                      n119 = property on="Select Pen Attributes" class="Clust (strict)"() -> ("Controls[]"=w365:refnum<vi>[])  [unwired: 2 in, 2 out]
                      n120 = case shown="\"Manual Mode\"" w366 {
                        tunnel: w365 -> [w370 w371 w375 w379 w383 w387 w391 w395]
                        tunnel: "Select Pen Attributes" -> [_ _ _ _ _ _ _ _]
                        frame "Manual Mode" {
                          # "All attributes are valid for this\noperation."
                          n121 = Index Array "Index Array"(array=w370, index=1) -> (element=w368:refnum<vi>)
                          n122 = property on="Property Node" class="Ctl"(reference=w368, "Disabled"=u8 0) -> ()  [unwired: 1 in, 2 out]
                        }
                        frame "Back Up" {
                          # "All attributes are valid for this\noperation."
                          n123 = Index Array(array=w371, index=1) -> (element=w373:refnum<vi>)
                          n124 = property class="Ctl"(reference=w373, "Disabled"=u8 0) -> ()  [unwired: 1 in, 2 out]
                        }
                        frame "Tug Off" {
                          # "All attributes are valid for this\noperation."
                          n125 = Index Array "Index Array"(array=w375, index=1) -> (element=w377:refnum<vi>)
                          n126 = property on="Property Node" class="Ctl"(reference=w377, "Disabled"=u8 0) -> ()  [unwired: 1 in, 2 out]
                        }
                        frame "Left Wall Follow" {
                          # "All attributes are valid for this\noperation."
                          n127 = Index Array "Index Array"(array=w379, index=1) -> (element=w381:refnum<vi>)
                          n128 = property on="Property Node" class="Ctl"(reference=w381, "Disabled"=u8 0) -> ()  [unwired: 1 in, 2 out]
                        }
                        frame "Goto WayPoint" {
                          # "All attributes are valid for this\noperation."
                          n129 = Index Array "Index Array"(array=w383, index=1) -> (element=w385:refnum<vi>)
                          n130 = property on="Property Node" class="Ctl"(reference=w385, "Disabled"=u8 0) -> ()  [unwired: 1 in, 2 out]
                        }
                        frame "Circle" {
                          # "All attributes are valid for this\noperation."
                          n131 = Index Array "Index Array"(array=w387, index=1) -> (element=w389:refnum<vi>)
                          n132 = property on="Property Node" class="Ctl"(reference=w389, "Disabled"=u8 0) -> ()  [unwired: 1 in, 2 out]
                        }
                        frame "Right Wall Follow" {
                          # "All attributes are valid for this\noperation."
                          n133 = Index Array "Index Array"(array=w391, index=1) -> (element=w393:refnum<vi>)
                          n134 = property on="Property Node" class="Ctl"(reference=w393, "Disabled"=u8 0) -> ()  [unwired: 1 in, 2 out]
                        }
                        frame "Hunt" {
                          # "All attributes are valid for this\noperation."
                          n135 = Index Array "Index Array"(array=w395, index=1) -> (element=w397:refnum<vi>)
                          n136 = property on="Property Node" class="Ctl"(reference=w397, "Disabled"=u8 0) -> ()  [unwired: 1 in, 2 out]
                        }
                      }
                      n137 = local read "initialized MDF"() -> (w363:T4)
                    }
                    event "MissionDefFile": Mouse Up {
                      # "When the user is finished drawing, we complete the operation."
                      # "Finished Drawing"
                      n138 = event-data() -> ()  [unwired: 1 in, 3 out]
                      n139 = local write "Draw??"(FALSE ("Draw??")) -> ()
                      n140 = local read "initialized MDF"() -> (w400:T4)
                    }
                  }
                  "MissionDefFile" <- w273
                  "MDF_Original" <- w271
                  n141 = call "UpdateMDF.vi"("Index"=0, "MDF_In"=w271) -> ("MDF_Out"=→"MDF":T4)  [unwired: 9 in]
                }
                n142 = Wait (ms)(milliseconds to wait=u32 200) -> ()  [unwired: 1 out]
                "Way Point Index" <- 0 ("Boundary Point Index")
              }
              frame #1 {
                w404 = T1."AutoMode" ("Tab")
                # "Force \nnext \ncase\nto  be\nAutoMode"
                n143 = local write "Tab"(w404) -> ()
                n144 = local write "Exit Planning"(FALSE ("Exit Planning")) -> ()
              }
            }
          }
          frame "ManualMode" {
            # "Removing map shift register\nfixed memory leak?"
            # "Manual Steering by dashboard heading steering wheel\nand by speed slider"
            # "This mode lets \noperator directly\ndrive robot via\nthe ManualMode\ntabbed interface"
            n145 = while {
              shift-right: [w434] -> _
              shift-left: _ -> [w433]
              tunnel: w408 -> [w426]
              shift-right: [w423] -> _
              shift-left: _ -> [w422]
              tunnel: w406 -> [w420]
              stop <- w432 stop-if-true
              # "WhereAmI?"
              n146 = Get Date/Time In Seconds "GetMiissionCurrentTime"() -> (seconds since 1Jan1904=w427:timestamp)
              n147 = call "WhereForebrainPerception.vi"("Where? Midbrain"="WhereAmI?FromBase") -> ("Where? Forebrain"=→"Where? Manual":T6, "(xr,yr)"=w423:cluster{"X":dbl, "Y":dbl}, "Direction"=w412:dbl)  [unwired: 3 in, 1 out]
              "(xr,yr)" <- w423
              n148 = local read "ManualModeStop"() -> (w432:bool)
              n149 = To Double Precision Float(number=w427) -> (double precision float=w428:dbl)
              n150 = Greater Or Equal?(x=w412, y=181.0) -> (x >= y?=w417:bool)
              n151 = local read "Manual Heading"() -> (w424:i16)
              n152 = Subtract(x=w428, y=w426) -> (x-y=w429:dbl)
              n153 = Not(x=w433) -> (.not. x?=w434:bool)
              n154 = call "DrawRobot.vi"("(xr,yr) old"=w422, "(xr,yr) new"=w423, "2D Picture"=w420) -> ("new picture"=→"ManualMissionMap":picture)
              n155 = Divide(x=w429, y=60.0) -> (x/y=w431:dbl)
              "MissionTime" <- w431
              n156 = Subtract(x=w412, y=360.0) -> (x-y=w415:dbl)
              n157 = shared-variable "My Computer\\RobotBrainExLibrary.lvlib\\MissionTime"(w431) -> ()  [unwired: 1 in, 1 out]
              n158 = Select(t=w415, s=w417, f=w412) -> (s? t:f=w414:dbl)
              n159 = Bundle("Direction"=w414, "Manual Heading"=w424) -> (→"Heading":cluster{"Direction":dbl, "Manual Heading":i16})  [unwired: 1 in]
              n160 = Wait Until Next ms Multiple(millisecond multiple=u32 100 ("milliseconds to wait")) -> ()  [unwired: 1 out]
              "Where? 2" <- w433
            }
            n161 = while {
              shift-right: [w441] -> _
              shift-left: _ -> [w442]
              stop <- "ManualModeStop" stop-if-true
              # "WhatIsAroundMe?"
              n162 = local read "WhatAroundMeMap?"() -> (w436:cluster{"T":dbl, "Range":dbl, "Bearing":dbl}[])
              n163 = call "ProcessLidarData.vi"("WhatAroundMe?MM"=w436) -> ("Collision"=w437:bool, "data array [mag, phase (deg)]"=w438:cluster{"magnitude":dbl, "phase":dbl}[])
              "CollisionLight" <- w437
              n164 = Not(x=w442) -> (.not. x?=w441:bool)
              "MWhat?" <- w441
              n165 = call "SimLIDARPlot.vi"("data array [mag, phase (deg)]"=w438) -> ("SONAR"=→"ManualModeMapDAR":picture)  [unwired: 1 in]
              n166 = case shown="True" w437 {
                frame False {
                  # "No \nBeep"
                }
                frame True {
                  n167 = call <vilib>:"Beep.vi"("use system alert? (T)"=TRUE, "duration (msec)"=u32 1000, "frequency (Hz)"=u32 900) -> ()  [unwired: 9 in]
                }
              }
              n168 = Wait Until Next ms Multiple(millisecond multiple=u32 100 ("milliseconds to wait")) -> ()  [unwired: 1 out]
            }
            n169 = while {
              shift-right: [w465] -> _
              shift-left: _ -> [w464]
              stop <- w463 stop-if-true
              # "HowAmI?"
              n170 = local read "Battery\nVolts"() -> (w462:i16)
              n171 = local read "ManualModeStop"() -> (w463:bool)
              n172 = Not(x=w464) -> (.not. x?=w465:bool)
              n173 = Divide(x=w462, y=i16 1000) -> (x/y=→"Battery":dbl)
              n174 = Wait Until Next ms Multiple(millisecond multiple=u32 100 ("milliseconds to wait")) -> ()  [unwired: 1 out]
              "How? 2" <- w464
            }
            n175 = while {
              shift-right: [w459] -> _
              shift-left: _ -> [w458]
              stop <- w457 stop-if-true
              # "ForebrainAct"
              n176 = local read "E-Stop"() -> (w455:bool)
              n177 = local read "ManualModeStop"() -> (w457:bool)
              n178 = Select(t=0.0, s=w455, f="Manual Vel") -> (s? t:f=w452:dbl)
              n179 = To Word Integer(number=w452) -> (16bit integer=w450:i16)
              "Speed" <- w450
              n180 = local read "Send String"() -> (→"Send String to NXT":string)
              n181 = To Word Integer(number="Behavior Command") -> (16bit integer=w447:i16)
              n182 = local write "Mode"(w447) -> ()
              n183 = local write "Desired \nVelocity"(w450) -> ()
              n184 = local write "Local\nHeading"("Manual Heading") -> ()
              n185 = Not(x=w458) -> (.not. x?=w459:bool)
              n186 = Wait Until Next ms Multiple(millisecond multiple=u32 50 ("milliseconds to wait")) -> ()  [unwired: 1 out]
              "ActManual" <- w458
            }
            n187 = local read "ManualModeStop"() -> (w409:bool)
            n188 = case shown="True" w409 {
              tunnel: [TRUE ("s") w469] -> w411
              tunnel: [T1."ManualMode" ("Tab") w470] -> w410
              frame False {
              }
              frame True {
                # "Debounce tab for clean transition"
                n189 = flat-sequence {
                  tunnel: [w476] -> w470
                  tunnel: [TRUE ("s")] -> w469
                  frame #0 {
                    n190 = Wait (ms)(milliseconds to wait=u32 100) -> ()  [unwired: 1 out]
                  }
                  frame #1 {
                    w476 = T1."Startup&Shutdown" ("Tab")
                    # "Turn off\nVelocity\non \nExit"
                    n191 = local write "ManualModeStop"(FALSE ("ManualModeStop")) -> ()
                    n192 = local write "Desired \nVelocity"(i16 0 ("Desired \nVelocity")) -> ()
                    n193 = local write "Local\nHeading"(i16 0 ("Local\nHeading")) -> ()
                    n194 = local write "Mode"(i16 0 ("Mode")) -> ()
                    n195 = local write "Tab"(w476) -> ()
                  }
                }
              }
            }
          }
          frame "AutoMode" {
            n196 = flat-sequence {
              tunnel: w484 -> [_]
              tunnel: [w487] -> w482
              tunnel: w481 -> [w487]
              tunnel: w480 -> [w486]
              tunnel: [w486] -> w479
              tunnel: w478 -> [_]
              tunnel: w482 -> [w494]
              tunnel: w479 -> [w492]
              tunnel: [w569] -> w485
              tunnel: [FALSE ("s")] -> w483
              frame #0 {
                # "Run Robot\nbased on\nmission\ndefinition\nfile"
                n197 = local write "AutoMissionMap"(w486) -> ()
                n198 = while {
                  shift-right: [w490] -> _
                  shift-left: _ -> [w489]
                  stop <- "RunAutoMode" continue-if-true
                  # "Wait for Run\nbutton press\nbefore\nturning on\nAutoMode\nCode"
                  n199 = Not(x=w489) -> (.not. x?=w490:bool)
                  n200 = Wait Until Next ms Multiple(millisecond multiple=u32 100 ("milliseconds to wait")) -> ()  [unwired: 1 out]
                  "Ready" <- w489
                }
              }
              frame #1 {
                n201 = while {
                  shift-right: [w540] -> _
                  shift-left: _ -> [w531]
                  tunnel: w494 -> [w535]
                  shift-right: [w533] -> _
                  shift-left: _ -> [w534]
                  tunnel: w492 -> [w526]
                  stop <- w530 stop-if-true
                  # "WhereAmI?"
                  n202 = local read "WhereAmI?FromBase"() -> (w525:T6)
                  n203 = Get Date/Time In Seconds "GetMiissionCurrentTime"() -> (seconds since 1Jan1904=w536:timestamp)
                  n204 = call "WhereForebrainPerception.vi"("Where? Midbrain"=w525) -> ("(xr,yr)"=w533:cluster{"X":dbl, "Y":dbl}, "Direction"=w519:dbl)  [unwired: 3 in, 2 out]
                  "Robot Position" <- w533
                  n205 = local read "RunAutoMode"() -> (w530:bool)
                  n206 = Greater Or Equal?(x=w519, y=181.0) -> (x >= y?=w523:bool)
                  n207 = To Double Precision Float(number=w536) -> (double precision float=w537:dbl)
                  n208 = Subtract(x=w537, y=w535) -> (x-y=w538:dbl)
                  n209 = Not(x=w531) -> (.not. x?=w540:bool)
                  n210 = call "DrawRobot.vi"("(xr,yr) old"=w534, "(xr,yr) new"=w533, "2D Picture"=w526) -> ("new picture"=→"AutoMissionMap":picture)
                  n211 = local read "SteerAngle"() -> (w528:dbl)
                  n212 = Divide(x=w538, y=60.0) -> (x/y=w532:dbl)
                  "MissionTimeAuto" <- w532
                  n213 = Subtract(x=w519, y=360.0) -> (x-y=w521:dbl)
                  n214 = Select(t=w521, s=w523, f=w519) -> (s? t:f=w520:dbl)
                  n215 = shared-variable "My Computer\\RobotBrainExLibrary.lvlib\\MissionTime"(w532) -> ()  [unwired: 1 in, 1 out]
                  n216 = Bundle("Direction"=w520, "SteerAngle"=w528) -> (→"A Heading":cluster{"Direction":dbl, "SteerAngle":dbl})  [unwired: 1 in]
                  n217 = Wait Until Next ms Multiple(millisecond multiple=u32 50 ("milliseconds to wait")) -> ()  [unwired: 1 out]
                  "Where?" <- w531
                }
                n218 = while {
                  shift-right: [w559] -> _
                  shift-left: _ -> [w558]
                  shift-right: [w554] -> _
                  shift-left: 0.0 ("SteerAngle") -> [w553]
                  stop <- w561 stop-if-true
                  # "needs to put out heading in local coordinates"
                  # "Think"
                  n219 = Not(x=w558) -> (.not. x?=w559:bool)
                  n220 = Or(x="Pause", y="E-Stop") -> (x .or. y?=w543:bool)
                  n221 = local read "WhereAmI?FromBase"() -> (w557:T6)
                  n222 = local read "WhatAroundMeMap?"() -> (w556:cluster{"T":dbl, "Range":dbl, "Bearing":dbl}[])
                  n223 = local read "MDF"() -> (w545:T4)
                  n224 = call "GotoWaypoint.vi"("InhibitIn"=w543, "CurrentSteerAngle"=w553, "WhatAroundMe? Clean"=w556, "WhereAmI? Clean"=w557, "MDF In"=w545) -> ("BehCom"=→"Current Behavior":T7, "MDF Out"=w548:T4, "ActCommand"=→"WayPointAct":dbl[], "Vel"=→"A Speed":dbl, "SteerAngle"=w554:dbl)  [unwired: 1 in, 1 out]
                  "SteerAngle" <- w554
                  n225 = local write "MDF"(w548) -> ()
                  n226 = local read "RunAutoMode"() -> (w561:bool)
                  n227 = local read "MDF_Original"() -> (w551:T4)
                  n228 = local read "MDF"() -> (w550:T4)
                  n229 = Select(t=w551, s="Rerun MDF", f=w550) -> (s? t:f=w547:T4)
                  n230 = local write "MDF"(w547) -> ()
                  n231 = Wait Until Next ms Multiple(millisecond multiple=u32 50 ("milliseconds to wait")) -> ()  [unwired: 1 out]
                  "Neo-C" <- w558
                }
                n232 = while {
                  shift-right: [w512] -> _
                  shift-left: _ -> [w514]
                  stop <- w511 stop-if-true
                  # "WhatIsAroundMe?"
                  n233 = local read "WhatAroundMeMap?"() -> (w508:cluster{"T":dbl, "Range":dbl, "Bearing":dbl}[])
                  n234 = call "ProcessLidarData.vi"("WhatAroundMe?MM"=w508) -> ("Collision"=w509:bool, "data array [mag, phase (deg)]"=w513:cluster{"magnitude":dbl, "phase":dbl}[])
                  "CollisionLight 2" <- w509
                  n235 = local read "RunAutoMode"() -> (w511:bool)
                  n236 = call "SimLIDARPlot.vi"("data array [mag, phase (deg)]"=w513) -> ("SONAR"=→"AutoModeLIDAR":picture)  [unwired: 1 in]
                  n237 = Not(x=w514) -> (.not. x?=w512:bool)
                  "What?" <- w512
                  n238 = case shown="True" w509 {
                    frame False {
                      # "No \nBeep"
                    }
                    frame True {
                      n239 = call <vilib>:"Beep.vi"("use system alert? (T)"=TRUE, "duration (msec)"=u32 1000, "frequency (Hz)"=u32 900) -> ()  [unwired: 9 in]
                    }
                  }
                  n240 = Wait Until Next ms Multiple(millisecond multiple=u32 50 ("milliseconds to wait")) -> ()  [unwired: 1 out]
                }
                n241 = while {
                  shift-right: [w506] -> _
                  shift-left: _ -> [w505]
                  stop <- w504 stop-if-true
                  # "HowAmI?"
                  n242 = local read "Battery\nVolts"() -> (w502:i16)
                  n243 = local read "RunAutoMode"() -> (w504:bool)
                  n244 = Not(x=w505) -> (.not. x?=w506:bool)
                  n245 = Divide(x=w502, y=i16 1000) -> (x/y=→"AutoBattery":dbl)
                  n246 = Wait Until Next ms Multiple(millisecond multiple=u32 80 ("milliseconds to wait")) -> ()  [unwired: 1 out]
                  "How?" <- w505
                }
                n247 = while {
                  shift-right: [w499] -> _
                  shift-left: _ -> [w498]
                  stop <- w497 stop-if-true
                  # "calculate desired heading.vi"
                  # "see calc desired\nheading"
                  # "convert to \noutputtin\nDesired v and\nlocal heading"
                  # "chnage arbiter to be -180 to 180"
                  # "Note:\nadd other beh to\narbiter"
                  # "ForebrainAct"
                  n248 = local read "WayPointAct"() -> (w496:dbl[])
                  n249 = local read "RunAutoMode"() -> (w497:bool)
                  n250 = Not(x=w498) -> (.not. x?=w499:bool)
                  n251 = call "ForebrainArbiter.vi"("WaypointInput"=w496) -> ("ForebrainActCom"=w495:dbl[])  [unwired: 14 in]
                  n252 = shared-variable "My Computer\\RobotBrainExLibrary.lvlib\\ActCommand"(w495) -> ()  [unwired: 1 in, 1 out]
                  n253 = Wait Until Next ms Multiple(millisecond multiple=u32 50 ("milliseconds to wait")) -> ()  [unwired: 1 out]
                  "Act" <- w498
                }
              }
              frame #2 {
                w569 = T1."Startup&Shutdown" ("Tab")
                # "Set robot Vel to 0"
                # "Reset latched run\nswitch"
                # "Force control to\nShutdown Case"
                n254 = shared-variable "My Computer\\RobotBrainExLibrary.lvlib\\ForebrainCom"(T8 {"VelCom"=0.0, "BehCom"=enum."OpenFieldTransit"} ("ForebrainCom")) -> ()  [unwired: 1 in, 1 out]
                n255 = local write "RunAutoMode"(TRUE ("RunAutoMode")) -> ()
                n256 = Initialize Array(0.0 ("element"), 90 ("dimension size")) -> (w565:dbl[])
                n257 = shared-variable "My Computer\\RobotBrainExLibrary.lvlib\\ActCommand"(w565) -> ()  [unwired: 1 in, 1 out]
                n258 = shared-variable "My Computer\\RobotBrainExLibrary.lvlib\\Xstart"(200.0 ("Xstart")) -> ()  [unwired: 1 in, 1 out]
                n259 = shared-variable "My Computer\\RobotBrainExLibrary.lvlib\\Ystart"(400.0 ("Ystart")) -> ()  [unwired: 1 in, 1 out]
                n260 = local write "Tab"(w569) -> ()
              }
            }
          }
          frame "Documentation" {
            # "Add:\n1) Blinking lights in each loop to show that they are running"
            # "This mode is just a static data flow picture of the ForeBrain"
            n261 = Wait (ms)(milliseconds to wait=u32 500) -> ()  [unwired: 1 out]
          }
          frame "DebugTHINK" {
            w579 = T1."Startup&Shutdown" ("Tab")
            # "Add:\n1) a button for each midbrain behavior to help in debugging\n2) graph of \"neural\" arbiter brain waves for each actuator\n3) a button for each forebrain behavior"
            # "Put code here in place of delay"
            # "Sends Tab Control\nback to Startup\ncase"
            n262 = Wait (ms)(milliseconds to wait=u32 5000) -> ()  [unwired: 1 out]
            n263 = local write "Tab"(w579) -> ()
          }
        }
        n264 = Not(x=w165) -> (.not. x?=w148:bool)
        "Robot Live" <- w148
      }
      n265 = while {
        tunnel: w56 -> [w132]
        tunnel: w55 -> [w131]
        tunnel: [w130] -> w53
        tunnel: [w129] -> w54
        shift-right: [w123] -> _
        shift-left: _ -> [w122]
        stop <- w133 continue-if-true
        w135 = 250  # timeout
        # "Finds and displays tugs position"
        # "runs continuously till program stops"
        # "Comminications with Base Station"
        # "receive string"
        # "If time out, post timeout and\nremove the timeout error"
        # "Read data from the port."
        n266 = Wait Until Next ms Multiple(millisecond multiple=u32 1) -> ()  [unwired: 1 out]
        n267 = UDP Read(connection ID=w132, timeout ms (25000)=w135, 8:w131) -> (data out=w124:string, error out=w136:errorcluster, 3:w129:refnum<k16>)  [unwired: 1 in, 2 out]
        n268 = local write "Base Station data rec'd"(w124) -> ()
        n269 = Unbundle By Name(w136) -> ("code"=w139:i32)
        n270 = Equal?(x=w139, y=56) -> (x = y?=w137:bool)
        "BS Time Out?" <- w137
        n271 = case shown="True" w137 {
          tunnel: [w146 errorcluster {"status"=FALSE, "code"=0, "source"=""} ("error out")] -> w130
          tunnel: w136 -> [w146 _]
          frame False {
          }
          frame True {
          }
        }
        n272 = call "PC parse the data.vi"("Nav String"=w124, "Tug"="Tug letter") -> ("Buoy locations"=w128:cluster{"regular expression":string, i32, i32}[], "Tug Location"=w126:T13, "Valid?"=w127:bool)  [unwired: 1 out]
        "Valid ?" <- w127
        n273 = local write "Buoy locations"(w128) -> ()
        n274 = case shown="True" w127 {
          tunnel: w126 -> [_ w145]
          frame False {
            # "No \nchange"
          }
          frame True {
            # "New values from BaseStation"
            n275 = shared-variable "My Computer\\RobotBrainExLibrary.lvlib\\MissionTime"() -> (w144:dbl)  [unwired: 1 in, 1 out]
            n276 = Unbundle(w145) -> (w143:i32, w142:i32, w141:i32)  [unwired: 1 out]
            n277 = local write "Tug X"(w143) -> ()
            n278 = local write "Tug Y"(w142) -> ()
            n279 = local write "Tug H"(w141) -> ()
            n280 = Bundle(w144, w143, w142, w141) -> (w140:cluster{dbl, i32, i32, i32})  [unwired: 1 in]
            n281 = local write "WhereAmI?FromBase"(w140) -> ()
          }
        }
        n282 = local read "RunRobot"() -> (w133:bool)
        n283 = Not(x=w122) -> (.not. x?=w123:bool)
        "udp rate" <- w122
      }
      n284 = while {
        tunnel: w57 -> [_]
        stop <- w99 continue-if-true
        # "loop timimng \ncontrolled externally"
        # "embed in loop to left latter"
        # "Send commands to NXT"
        n285 = local read "Mode"() -> (w100:i16)
        n286 = local read "Desired \nVelocity"() -> (w101:i16)
        n287 = local read "Local\nHeading"() -> (w102:i16)
        n288 = Number To Decimal String(number=w100, width (-)=i16 2) -> (decimal integer string=w106:string)
        n289 = Number To Decimal String(number=w101, width (-)=i16 2) -> (decimal integer string=w105:string)
        n290 = Number To Decimal String(number=w102, width (-)=i16 4) -> (decimal integer string=w104:string)
        n291 = Concatenate Strings("$P", w106, w105, w104, "^") -> (w103:string)
        n292 = local read "RunRobot"() -> (w99:bool)
        n293 = local write "Send String"(w103) -> ()
      }
      n294 = while {
        tunnel: w57 -> [_]
        stop <- w76 continue-if-true
        # "Receive information from NXT"
        n295 = local read "String Received"() -> (w81:string)
        n296 = Wait Until Next ms Multiple(millisecond multiple=u32 100) -> ()  [unwired: 1 out]
        n297 = String Subset(string=w81, offset (0)=1, length (rest)=1 ("length (rest)")) -> (substring=w80:string)
        n298 = case shown="\"N\"" w80 {
          tunnel: w81 -> [_ w83]
          frame Default {
          }
          frame "N" {
            # "0-15"
            # "Parse command \"N\""
            n299 = String Subset(string=w83, offset (0)=2, length (rest)=4 ("length (rest)")) -> (substring=w94:string)
            n300 = String Subset(string=w83, offset (0)=6, length (rest)=3 ("length (rest)")) -> (substring=w90:string)
            n301 = String Subset(string=w83, offset (0)=9, length (rest)=2 ("length (rest)")) -> (substring=w86:string)
            n302 = Decimal String To Number(string=w94) -> (number=w97:i32)  [unwired: 2 in, 1 out]
            n303 = Decimal String To Number(string=w90) -> (number=w89:i32)  [unwired: 2 in, 1 out]
            n304 = Decimal String To Number(string=w86) -> (number=w87:i32)  [unwired: 2 in, 1 out]
            n305 = To Word Integer(number=w97) -> (16bit integer=w93:i16)
            n306 = To Word Integer(number=w89) -> (16bit integer=w88:i16)
            n307 = To Long Integer(number=w87) -> (32bit integer=w82:i32)
            n308 = local write "LidarDist"(w88) -> ()
            n309 = local write "Battery\nVolts"(w93) -> ()
            n310 = local write "IR Index"(w82) -> ()
          }
        }
        n311 = local read "RunRobot"() -> (w76:bool)
      }
      n312 = while {
        stop <- w75 continue-if-true
        # "Run Simulated MapDAR"
        n313 = local read "Tug X"() -> (w73:i32)
        n314 = local read "Tug Y"() -> (w72:i32)
        n315 = local read "Tug H"() -> (w71:i32)
        n316 = Bundle "Bundle"("Tug X"=w73, "Tug Y"=w72, "Tug H"=w71) -> (w74:cluster{"Tug X":i32, "Tug Y":i32, "Tug H":i32})  [unwired: 1 in]
        n317 = call "HindbrainLIDAR_Sim.vi"("SubPosition"=w74) -> ("WhatAroundMe?"=→"WhatAroundMeMap?":cluster{"T":dbl, "Range":dbl, "Bearing":dbl}[])  [unwired: 10 in]
        n318 = local read "RunRobot"() -> (w75:bool)
      }
    }
    frame #2 {
      # "Close XBee Radio"
      # "Close UDP port"
      # "Realease LIDAR\nMemory"
      # "Reset Run \nSwitch"
      # "Shutdown Robot"
      n319 = call "Pixel_LIDAR_Close.vi"("error in (no error) 2"=w585, "Image"=w586) -> ()  [unwired: 1 in]
      n320 = local write "RunRobot"(TRUE ("RunRobot")) -> ()
      n321 = call "XB PC Close.vi"("error in (no error)"=w583, "VISA resource name"=w584) -> ()
      n322 = UDP Close(connection ID=w582, 8:w581) -> ()  [unwired: 2 out]
      "error out" <- w583
    }
  }
